vi "file path create (host).vi"(11 "experiment name":string) -> (0 "error out":errorcluster, 2 "samples file":refnum<file>, 3 "csi file":refnum<file>)   [LabVIEW 2020]
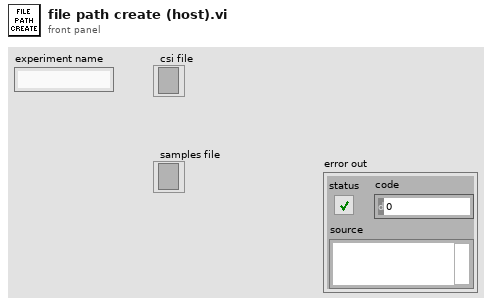
[diagram p1: front panel]
types:
  T1 = enum16{"open", "replace", "create", "open or create", "replace or create", "replace or create with confirmation"}
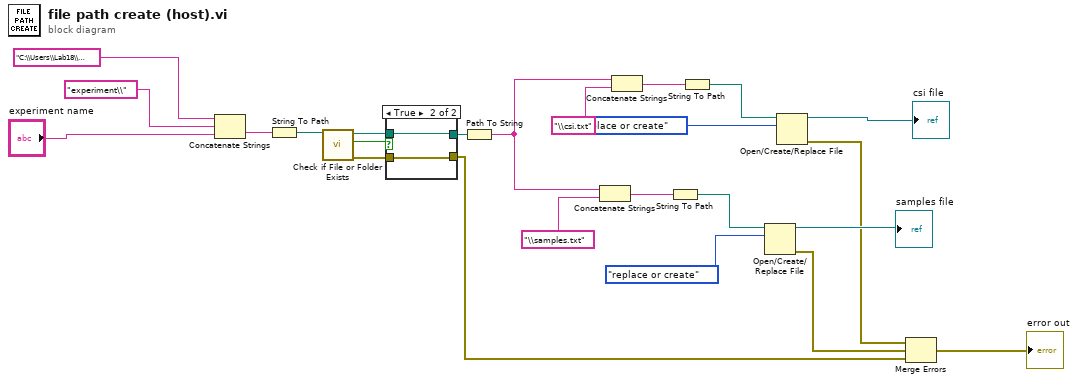
[diagram p0: block diagram]
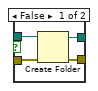
[diagram p2: hidden frame]
diagram:
  n1 = Concatenate Strings("C:\\Users\\Lab18\\Documents\\LabVIEW Data\\WiFi MUSIC\\", "experiment\\", "experiment name") -> (w14:string)
  n2 = String To Path(string=w14) -> (path=w4:path)
  n3 = call <vilib>:"Check if File or Folder Exists.vi"("path"=w4) -> ("error out"=w2:errorcluster, "file or folder exists?"=w1:bool, "dup path"=w3:path)  [unwired: 8 in]
  n4 = case shown="True" w1 {
    tunnel: [w28 w29] -> w15
    tunnel: [w27 w30] -> w7
    tunnel: w3 -> [w26 w29]
    tunnel: w2 -> [w25 w30]
    frame False {
      n5 = Create Folder(path (use dialog)=w26, error in=w25) -> (created path=w28:path, error out=w27:errorcluster)  [unwired: 1 in, 1 out]
    }
    frame True {
    }
  }
  n6 = Path To String(path=w15) -> (string=w22:string)
  n7 = Concatenate Strings(w22, "\\samples.txt") -> (w21:string)
  n8 = Concatenate Strings(w22, "\\csi.txt") -> (w17:string)
  n9 = String To Path(string=w21) -> (path=w19:path)
  n10 = String To Path(string=w17) -> (path=w13:path)
  n11 = Open/Create/Replace File(file path (use dialog)=w19, operation (0:open)=T1."replace or create") -> (refnum out=→"samples file":refnum<file>, error out=w6:errorcluster)  [unwired: 4 in, 1 out]
  n12 = Open/Create/Replace File(file path (use dialog)=w13, operation (0:open)=T1."replace or create") -> (refnum out=→"csi file":refnum<file>, error out=w5:errorcluster)  [unwired: 4 in, 1 out]
  n13 = Merge Errors(w5, w6, w7) -> (→"error out":errorcluster)
